vi "Finish.vi"   [LabVIEW 2014]
doc: "This VI is called just before exiting. It is expected to close I/O refnum, save collected data, etc."
uses:
  <vilib>/Rock Robotics/WPI/Joystick/WPI_JoystickGetSetRefNum.vi
  <vilib>/Rock Robotics/WPI/RobotDrive/WPI_RobotDriveGetSetRefNum.vi
  <vilib>/Rock Robotics/WPI/Ultrasonic/WPI_SonarMB1010AnalogRefNum Registry Get.vi
  <vilib>/Rock Robotics/WPI/Ultrasonic/WPI_SonarMB1010AnalogClose.vi
types:
  T1 = typedef "WPI_SonarMB1010AnalogDeviceRef.ctl" = cluster{"AIDeviceRef":T2, "Scaling factor (V/in)":dbl, "Average Bits":u8}
  T2 = typedef "WPI_AnalogChannelDevRef.ctl" = cluster{"DevStatus":errorcluster, "Controller":T3, "Analog Channel":T4}
  T3 = typedef "FPGA_TypedefAnalogModule.ctl" = enum16{"Controller 1"}
  T4 = typedef "FPGA_AIChannel.ctl" = enum8{"AI 0", "AI 1", "AI 2", "AI 3", "AI MXP 0", "AI MXP 1", "AI MXP 2", "AI MXP 3", "Invalid"}
  T5 = typedef "WPI_AccelerometerDevRef.ctl" = cluster{"DevStatus":errorcluster, "Controller":T3, "Scaling":T6, "Analog Channels":T7, "I2C Bus":T8, "SPI Bus":T9, "Accel Range":T10, "ADXL345 Axes":T11, "Handle":i32, "Device Address":u8, "Accel Type":enum16{"Analog", "ADXL345 I2C", "ADXL345 SPI", "Internal"}}
  T6 = typedef "WPI_AccelerometerScaling.ctl" = cluster{"Gain (VoltsPerG)":dbl, "Center Voltage":dbl}
  T7 = typedef "WPI_AccelerometerAnalogChannels.ctl" = cluster{"X-Axis":T4, "Y-Axis":T4, "Z-Axis":T4}
  T8 = typedef "i2c_bus.ctl" = enum16{"I2C On-Board", "I2C MXP", "Invalid"}
  T9 = typedef "spi_bus.ctl" = enum16{"SPI On-Board, CS0", "SPI On-Board, CS1", "SPI On-Board, CS2", "SPI On-Board, CS3", "SPI MXP", "Invalid"}
  T10 = typedef "ADXL345 Range.ctl" = u8
  T11 = typedef "WPI_AccelerometerADXL345 Axes.ctl" = cluster{"X-Axis":bool, "Y-Axis":bool, "Z-Axis":bool}
  T12 = typedef "WPI_SwitchDevRef.ctl" = cluster{"DevStatus":errorcluster, "DIO Channel":T13, "Controller":T14, "CntIndex":T15, "Normally Closed":bool}
  T13 = typedef "FPGA_DIOChannel.ctl" = enum8{"DIO 0", "DIO 1", "DIO 2", "DIO 3", "DIO 4", "DIO 5", "DIO 6", "DIO 7", "DIO 8", "DIO 9", "DIO MXP 0", "DIO MXP 1", "DIO MXP 2", "DIO MXP 3", "DIO MXP 4", "DIO MXP 5", "DIO MXP 6", "DIO MXP 7", "DIO MXP 8", "DIO MXP 9", "DIO MXP 10", "DIO MXP 11", "DIO MXP 12", "DIO MXP 13", "DIO MXP 14", "DIO MXP 15", "Invalid"}
  T14 = typedef "FPGA_TypedefDigitalModule.ctl" = enum16{"Controller 1"}
  T15 = typedef "FPGA_CounterCtrSystemIndex.ctl" = enum8{"Ctr 0", "Ctr 1", "Ctr 2", "Ctr 3", "Ctr 4", "Ctr 5", "Ctr 6", "Ctr 7", "Invalid"}
  T16 = typedef "WPI_MotorControlDeviceRef.ctl" = cluster{"DeviceStatus":errorcluster, "Type":T17, "PWM":cluster{"Controller":T14, "PWM Channel":T18, "DeadBand":T19}, "CAN":cluster{"Device Number":u8, "Control Mode":T20, "Semaphore":T21, "Max Vout":dbl, "TalonSRX Control Mode":T22}, "Invert":bool, "TransformRef":T23, "InvTransformRef":T23}
  T17 = typedef "WPI_MotorControlType.ctl" = enum16{"PWM", "CAN", "CANTalonSRX"}
  T18 = typedef "FPGA_DIOPWMChannel.ctl" = enum8{"PWM 0", "PWM 1", "PWM 2", "PWM 3", "PWM 4", "PWM 5", "PWM 6", "PWM 7", "PWM 8", "PWM 9", "PWM MXP 0", "PWM MXP 1", "PWM MXP 2", "PWM MXP 3", "PWM MXP 4", "PWM MXP 5", "PWM MXP 6", "PWM MXP 7", "PWM MXP 8", "PWM MXP 9", "Invalid"}
  T19 = typedef "WPI_PWMDeadband.ctl" = cluster{"Name":string, "maxPositivePwm":i32, "minPositivePwm":i32, "centerPwm":i32, "maxNegativePwm":i32, "minNegativePwm":i32, "angularRange":u16}
  T20 = typedef "WPI_CANJaguar_ControlMode.ctl" = enum8{"Percent VBus", "Current", "Speed", "Position", "Voltage"}
  T21 = typedef "Semaphore RefNum" = refnum<k1>
  T22 = typedef "WPI_CANTalonSRX_APIControlMode.ctl" = enum8{"Percent VBus", "Speed", "Position", "Slave", "Unchanged / Invalid"}
  T23 = typedef "WPI_PWMTransform_ConPane.ctl" = refnum<vi>
  T24 = typedef "WPI_PotentiometerDevRef.ctl" = cluster{"DevStatus":errorcluster, "Controller":T3, "Analog Channel":T4, "Invert Output":bool}
  T25 = typedef "WPI_JoystickDevRef.ctl" = cluster{"Device":T26}
  T26 = typedef "WPI_JoystickDeviceEnum.ctl" = enum16{"USB 0", "USB 1", "USB 2", "USB 3", "USB 4", "USB 5"}
  T27 = typedef "WPI_RobotDriveDevRef.ctl" = cluster{"DevStatus":errorcluster, "Motors[]":T16[], "Square Inputs":bool, "Max Output":dbl}
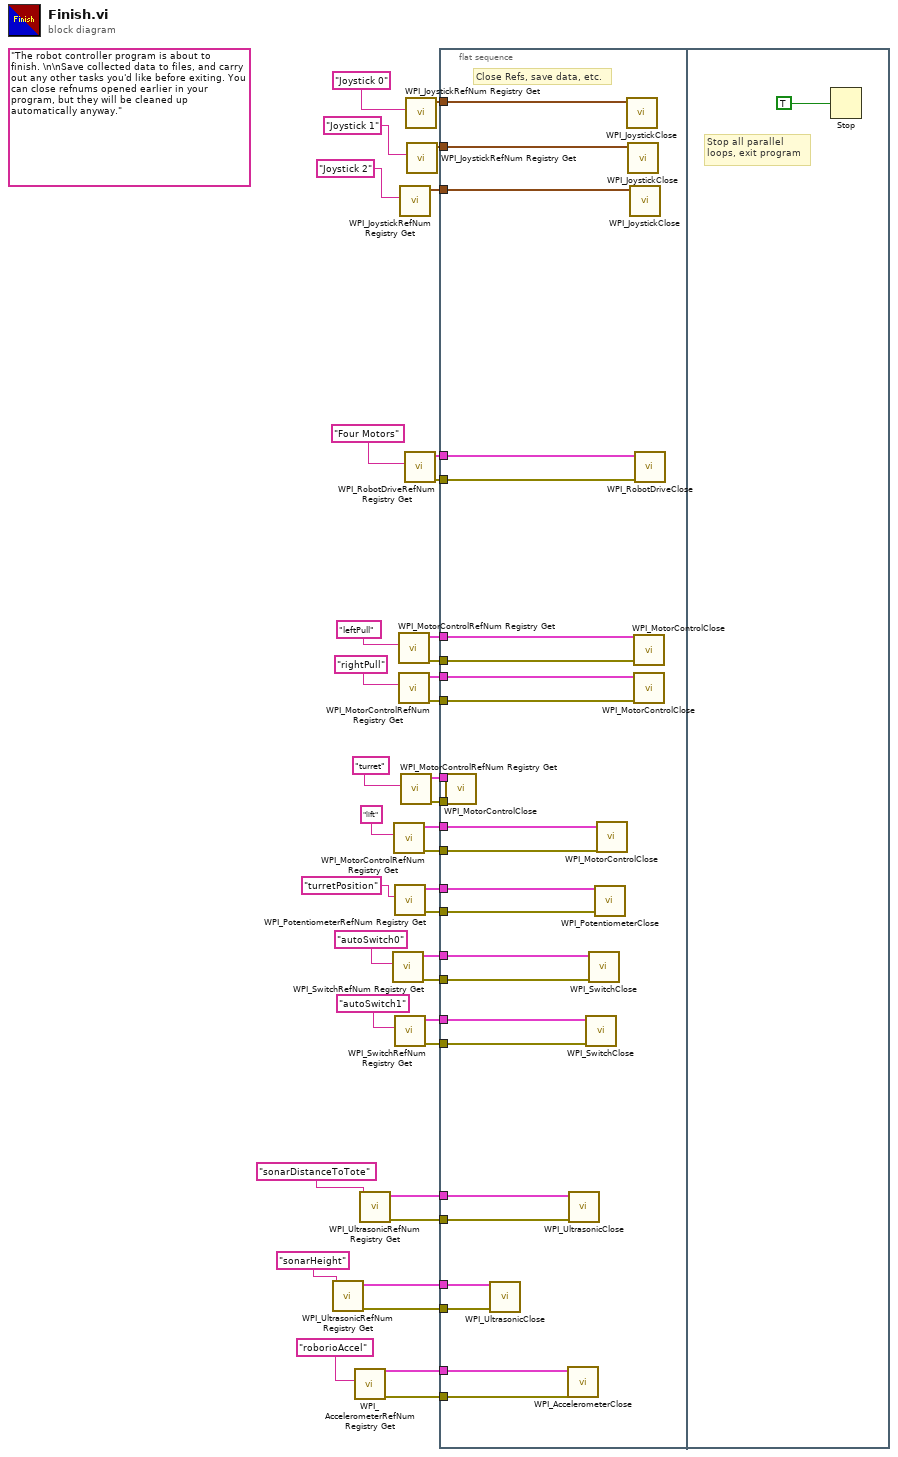
[diagram p0: block diagram]
diagram:
  (unwired) "The robot controller program is about to finish. \n\nSave collected data to files, and carry out any other tasks you'd like before exiting. You can close refnums opened earlier in your program, but they will be cleaned up automatically anyway."
  n1 = call-poly <vilib>:"WPI_UltrasonicRefNum Registry Get.vi"("refnum name"="sonarHeight") -> ("error out"=w1:errorcluster, "SonarMB1010AnalogDevRef"=w2:T1)  [unwired: 9 in]
  n2 = call <vilib>:"WPI_AccelerometerRefNum Registry Get.vi"("refnum name"="roborioAccel") -> ("error out"=w5:errorcluster, "AccelerometerDevRef"=w6:T5)  [unwired: 9 in]
  n3 = call-poly <vilib>:"WPI_UltrasonicRefNum Registry Get.vi"("refnum name"="sonarDistanceToTote") -> ("error out"=w7:errorcluster, "SonarMB1010AnalogDevRef"=w8:T1)  [unwired: 9 in]
  n4 = call <vilib>:"WPI_SwitchRefNum Registry Get.vi"("refnum name"="autoSwitch0") -> ("error out"=w14:errorcluster, "SwitchDevRef"=w15:T12)  [unwired: 9 in]
  n5 = call <vilib>:"WPI_MotorControlRefNum Registry Get.vi"("refnum name"="lift") -> ("error out"=w19:errorcluster, "MotorControlDevRef"=w20:T16)  [unwired: 9 in]
  n6 = call <vilib>:"WPI_PotentiometerRefNum Registry Get.vi"("refnum name"="turretPosition") -> ("error out"=w16:errorcluster, "PotDevRef"=w17:T24)  [unwired: 9 in]
  n7 = call <vilib>:"WPI_SwitchRefNum Registry Get.vi"("refnum name"="autoSwitch1") -> ("error out"=w10:errorcluster, "SwitchDevRef"=w11:T12)  [unwired: 9 in]
  n8 = call <vilib>:"WPI_MotorControlRefNum Registry Get.vi"("refnum name"="leftPull") -> ("error out"=w29:errorcluster, "MotorControlDevRef"=w30:T16)  [unwired: 9 in]
  n9 = call <vilib>:"WPI_MotorControlRefNum Registry Get.vi"("refnum name"="rightPull") -> ("error out"=w26:errorcluster, "MotorControlDevRef"=w27:T16)  [unwired: 9 in]
  n10 = call <vilib>:"WPI_JoystickRefNum Registry Get.vi"("refnum name"="Joystick 2") -> ("JoystickDevRef"=w32:T25)  [unwired: 1 in, 9 out]
  n11 = call <vilib>:"WPI_MotorControlRefNum Registry Get.vi"("refnum name"="turret") -> ("error out"=w23:errorcluster, "MotorControlDevRef"=w24:T16)  [unwired: 9 in]
  n12 = call <vilib>:"WPI_RobotDriveRefNum Registry Get.vi"("refnum name"="Four Motors") -> ("error out"=w31:errorcluster, "RobotDriveDevRef"=w37:T27)  [unwired: 1 in, 8 out]
  n13 = call <vilib>:"WPI_JoystickRefNum Registry Get.vi"("refnum name"="Joystick 0") -> ("JoystickDevRef"=w36:T25)  [unwired: 1 in, 9 out]
  n14 = call <vilib>:"WPI_JoystickRefNum Registry Get.vi"("refnum name"="Joystick 1") -> ("JoystickDevRef"=w35:T25)  [unwired: 1 in, 9 out]
  n15 = flat-sequence {
    tunnel: w37 -> [w64]
    tunnel: w36 -> [w63]
    tunnel: w35 -> [w62]
    tunnel: w32 -> [w61]
    tunnel: w31 -> [w60]
    tunnel: w30 -> [w59]
    tunnel: w29 -> [w58]
    tunnel: w27 -> [w57]
    tunnel: w26 -> [w56]
    tunnel: w24 -> [w55]
    tunnel: w23 -> [w54]
    tunnel: w20 -> [w53]
    tunnel: w19 -> [w52]
    tunnel: w17 -> [w51]
    tunnel: w16 -> [w50]
    tunnel: w15 -> [w49]
    tunnel: w14 -> [w48]
    tunnel: w11 -> [w47]
    tunnel: w10 -> [w46]
    tunnel: w8 -> [w45]
    tunnel: w7 -> [w44]
    tunnel: w6 -> [w43]
    tunnel: w5 -> [w42]
    tunnel: w2 -> [w41]
    tunnel: w1 -> [w40]
    frame #0 {
      # "Close Refs, save data, etc."
      n16 = call <vilib>:"WPI_MotorControlClose.vi"("error in (no error)"=w54, "MotorControlDevRef"=w55) -> ()  [unwired: 9 in, 1 out]
      n17 = call-poly <vilib>:"WPI_UltrasonicClose.vi"("error in"=w40, "SonarMB1010AnalogDevRef"=w41) -> ()  [unwired: 9 in, 1 out]
      n18 = call <vilib>:"WPI_AccelerometerClose.vi"("error in"=w42, "AccelerometerDevRef"=w43) -> ()  [unwired: 9 in, 1 out]
      n19 = call-poly <vilib>:"WPI_UltrasonicClose.vi"("error in"=w44, "SonarMB1010AnalogDevRef"=w45) -> ()  [unwired: 9 in, 1 out]
      n20 = call <vilib>:"WPI_SwitchClose.vi"("error in (no error)"=w46, "SwitchDevRef"=w47) -> ()  [unwired: 9 in, 1 out]
      n21 = call <vilib>:"WPI_SwitchClose.vi"("error in (no error)"=w48, "SwitchDevRef"=w49) -> ()  [unwired: 9 in, 1 out]
      n22 = call <vilib>:"WPI_PotentiometerClose.vi"("error in"=w50, "PotDevRef"=w51) -> ()  [unwired: 9 in, 1 out]
      n23 = call <vilib>:"WPI_MotorControlClose.vi"("error in (no error)"=w52, "MotorControlDevRef"=w53) -> ()  [unwired: 9 in, 1 out]
      n24 = call <vilib>:"WPI_JoystickClose.vi"("JoystickDevRef"=w63) -> ()  [unwired: 11 out]
      n25 = call <vilib>:"WPI_JoystickClose.vi"("JoystickDevRef"=w62) -> ()  [unwired: 11 out]
      n26 = call <vilib>:"WPI_JoystickClose.vi"("JoystickDevRef"=w61) -> ()  [unwired: 11 out]
      n27 = call <vilib>:"WPI_MotorControlClose.vi"("error in (no error)"=w58, "MotorControlDevRef"=w59) -> ()  [unwired: 9 in, 1 out]
      n28 = call <vilib>:"WPI_MotorControlClose.vi"("error in (no error)"=w56, "MotorControlDevRef"=w57) -> ()  [unwired: 9 in, 1 out]
      n29 = call <vilib>:"WPI_RobotDriveClose.vi"("error in (no error)"=w60, "RobotDriveDevRef"=w64) -> ()  [unwired: 10 out]
    }
    frame #1 {
      # "Stop all parallel\nloops, exit program"
      n30 = Stop(stop? (T)=TRUE ("Quit")) -> ()
    }
  }
